vi "DriveLoopQCP.vi"   [LabVIEW 2017]
uses:
  <userlib>/836-Library/System/QCP_V2/QCPSupportCode/QCP_GetDbl.vi
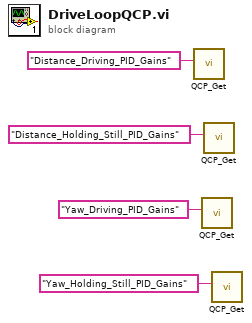
[diagram p0: block diagram]
diagram:
  n1 = call-poly <userlib>:"QCP_Get.vi"("Value Name"="Distance_Driving_PID_Gains") -> ()  [unwired: 8 in, 3 out]
  n2 = call-poly <userlib>:"QCP_Get.vi"("Value Name"="Yaw_Driving_PID_Gains") -> ()  [unwired: 8 in, 3 out]
  n3 = call-poly <userlib>:"QCP_Get.vi"("Value Name"="Distance_Holding_Still_PID_Gains") -> ()  [unwired: 8 in, 3 out]
  n4 = call-poly <userlib>:"QCP_Get.vi"("Value Name"="Yaw_Holding_Still_PID_Gains") -> ()  [unwired: 8 in, 3 out]
